vi "Send.vi"(8 "error in":errorcluster, 11 "Data":string="Send") -> (0 "error out":errorcluster)   [LabVIEW 2015, in "TCP.lvlib"]
uses:
  TCP.lvlib
  support/Message Queue/Enqueue Message (Single).vi
  support/Message Queue/Message Queue.lvlib
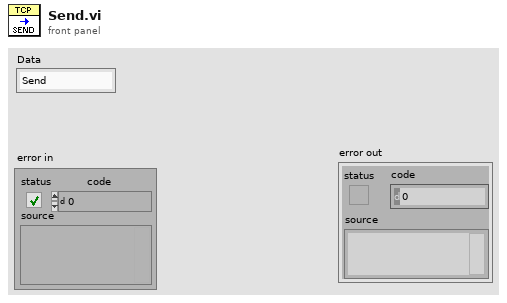
[diagram p1: front panel]
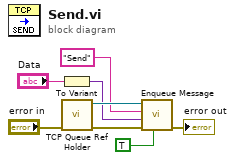
[diagram p0: block diagram]
diagram:
  n1 = To Variant(anything="Data") -> (Variant=w3:variant)
  n2 = call "TCP Queue Ref Holder.vi"("error in"="error in") -> ("error out"=w7:errorcluster, "Input Message Queue"=w5:refnum<queue>)  [unwired: 9 in]
  n3 = call-poly "Enqueue Message.vi"("Priority Message? (F)"=TRUE, "error in (no error)"=w7, "Message Data"=w3, "Message"="Send", "Message Queue"=w5) -> ("error out"=→"error out":errorcluster)  [unwired: 5 in, 1 out]
